vi "SMTP Email EUC To JIS.vi"(11 "text in":string) -> (3 "text out":string)   [LabVIEW 2012, in "NewNI_SMTPEmail.lvlib"]
uses:
  NewNI_SMTPEmail.lvlib
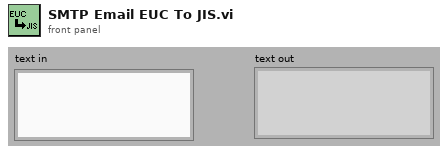
[diagram p1: front panel]
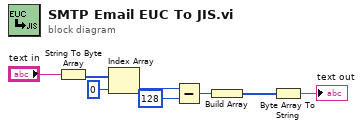
[diagram p0: block diagram]
diagram:
  n1 = String To Byte Array(string="text in") -> (unsigned byte array=w7:u8[])
  n2 = Index Array(array=w7, index=0) -> (element=w4:u8)
  n3 = Subtract(x=w4, y=u8 128) -> (x-y=w2:u8)
  n4 = Build Array(w2) -> (w1:u8[])
  n5 = Byte Array To String(unsigned byte array=w1) -> (string=→"text out":string)
